vi "Main.vi"(8 "error in (no error)":errorcluster) -> (0 "error out":errorcluster, 3 "007 Data":T2)   [LabVIEW 2015]
uses:
  007 Data.ctl
  Suit Enum.ctl
panel:
  in  "Bypass wait loop":bool
  out "Suit Score 2":dbl
  out "Suit Score 1":dbl
  out "Suit Card 2":T1
  out "Suit Card 1":T1
  out "Waiting in loop for 007 = yellow":bool
  out "My Turn?":bool
  in  "SS Image Path":path=path "c:/PokerSS/SS.png"
  out "All Players Money":string[](array[string])
  out "All Players Names":string[](array[string])
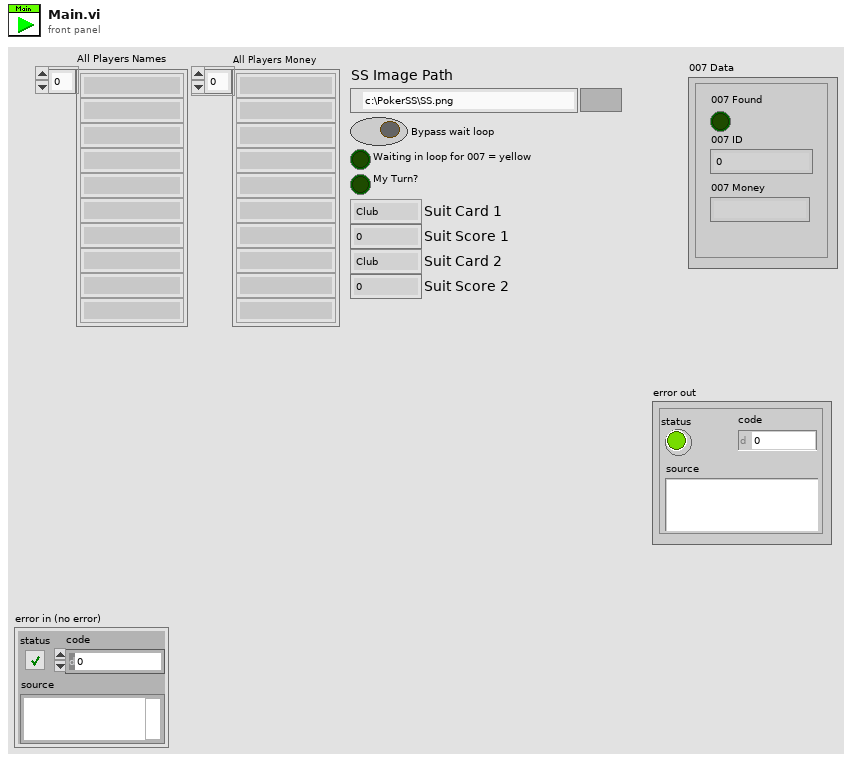
[diagram p1: front panel]
types:
  T1 = typedef "Suit Enum.ctl" = enum16{"Club", "Diamond", "Heart", "Spade", "Unknown"}
  T2 = typedef "007 Data.ctl" = cluster{"007 ID":dbl, "007 Found":bool, "007 Money":string}
  T3 = cluster{"Global Rectangle":i32[], "Contours":cluster{"ID":enum32{"External", "Internal"}, "Type":u32, "Coordinates":i32[]}[]}
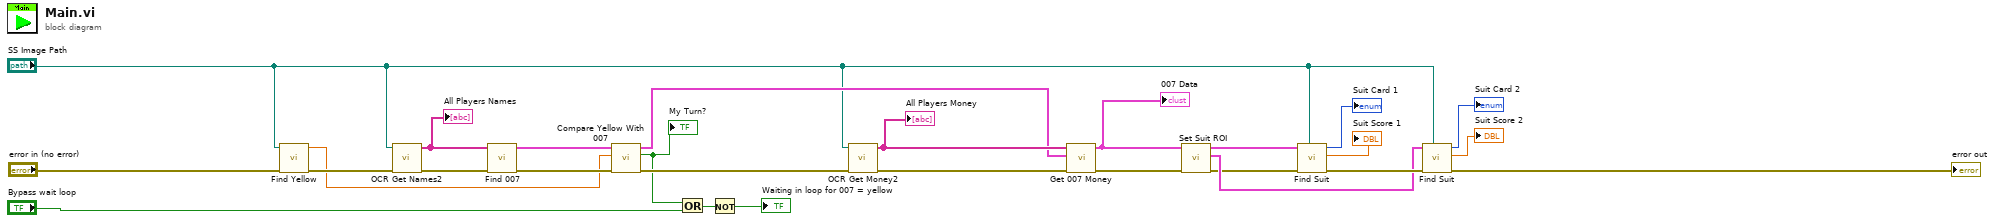
[diagram p0: block diagram]
diagram:
  n1 = call "Find Yellow.vi"("error in"="error in (no error)", "SS File Path"="SS Image Path") -> ("error out"=w22:errorcluster, "Yellow Player"=w18:dbl)  [unwired: 6 in]
  n2 = call "OCR Get Names2.vi"("error in"=w22, "SS Path"="SS Image Path") -> ("Error Out"=w23:errorcluster, "All Players Names"=w21:string[])  [unwired: 7 in]
  "All Players Names" <- w21
  n3 = call "Find 007.vi"("Error In"=w23, "Player Names"=w21) -> ("Error Out"=w20:errorcluster, "007 Data"=w19:T2)  [unwired: 8 in]
  n4 = call "Compare Yellow With 007.vi"("Error In"=w20, "Yellow Player"=w18, "007 Data"=w19) -> ("Error Out"=w27:errorcluster, "007s Turn"=w17:bool, "007 Data Out"=w24:T2)  [unwired: 6 in]
  "My Turn?" <- w17
  n5 = Or(x=w17, y="Bypass wait loop") -> (x .or. y?=w16:bool)
  n6 = Not(x=w16) -> (.not. x?=→"Waiting in loop for 007 = yellow":bool)
  n7 = call "OCR Get Money2.vi"("error in"=w27, "Path"="SS Image Path") -> ("error out"=w15:errorcluster, "Player Money"=w26:string[])  [unwired: 7 in]
  "All Players Money" <- w26
  n8 = call "Get 007 Money.vi"("Error In"=w15, "007 Data"=w24, "Player Money"=w26) -> ("Error Out"=w3:errorcluster, "007 Data Out"=w14:T2)  [unwired: 7 in]
  "007 Data" <- w14
  n9 = call "Set Suit ROI.vi"("Error In"=w3, "007 Data Out"=w14) -> ("Error Out"=w2:errorcluster, "ROI 2nd Card"=w8:T3, "ROI 1st Card"=w12:T3)  [unwired: 7 in]
  n10 = call "Find Suit.vi"("SS Path"="SS Image Path", "error in (no error)"=w2, "ROI 1st Card"=w12) -> ("error out"=w10:errorcluster, "Suit Score"=→"Suit Score 1":dbl, "Suit of Card"=→"Suit Card 1":T1)  [unwired: 5 in]
  n11 = call "Find Suit.vi"("SS Path"="SS Image Path", "error in (no error)"=w10, "ROI 1st Card"=w8) -> ("error out"=→"error out":errorcluster, "Suit Score"=→"Suit Score 2":dbl, "Suit of Card"=→"Suit Card 2":T1)  [unwired: 5 in]
